vi "Collision test full.vi"(5 "Triangle to test":T1, 6 "Query triangles":T1[](array[typedef]), 7 "Octree for query triangles":T2[](array[typedef])) -> (0 "Collision point(s)":sgl[][](array[numeric]), 1 "Minimum separation vector\n(from test triangle)":sgl[](array[numeric]), 2 "Minimum separation":sgl, 3 "Indices of possible triangles":i32[](array[numeric]), 4 "Collision(s)?":bool)   [LabVIEW 2014]
doc: "This VI returns all the collision points between the test triangle and the query triangles, as well as the minimum separation vector and distance in the case of no collision."
uses:
  Typedefs/Triangle.ctl
  Typedefs/TreeNodeBox.ctl
  Typedefs/Quad.ctl
panel:
  # "PN 03/02/2015"
  # "Vertices"
  # "Edges"
  # "Unit normal"
  # "Edge unit normals"
  # "Vertices"
  # "Edges"
  # "Unit normal"
  # "Edge unit normals"
  # "Vertices"
  # "Edges"
  # "Unit normal"
  # "Edge unit normals"
  # "Vertices"
  # "Edges"
  # "Unit normal"
  # "Edge unit normals"
  # "Vertices"
  # "Edges"
  # "Unit normal"
  # "Edge unit normals"
  # "Vertices"
  # "Edges"
  # "Unit normal"
  # "Edge unit normals"
  # "Vertices"
  # "Edges"
  # "Unit normal"
  # "Edge unit normals"
  # "Vertices"
  # "Edges"
  # "Unit normal"
  # "Edge unit normals"
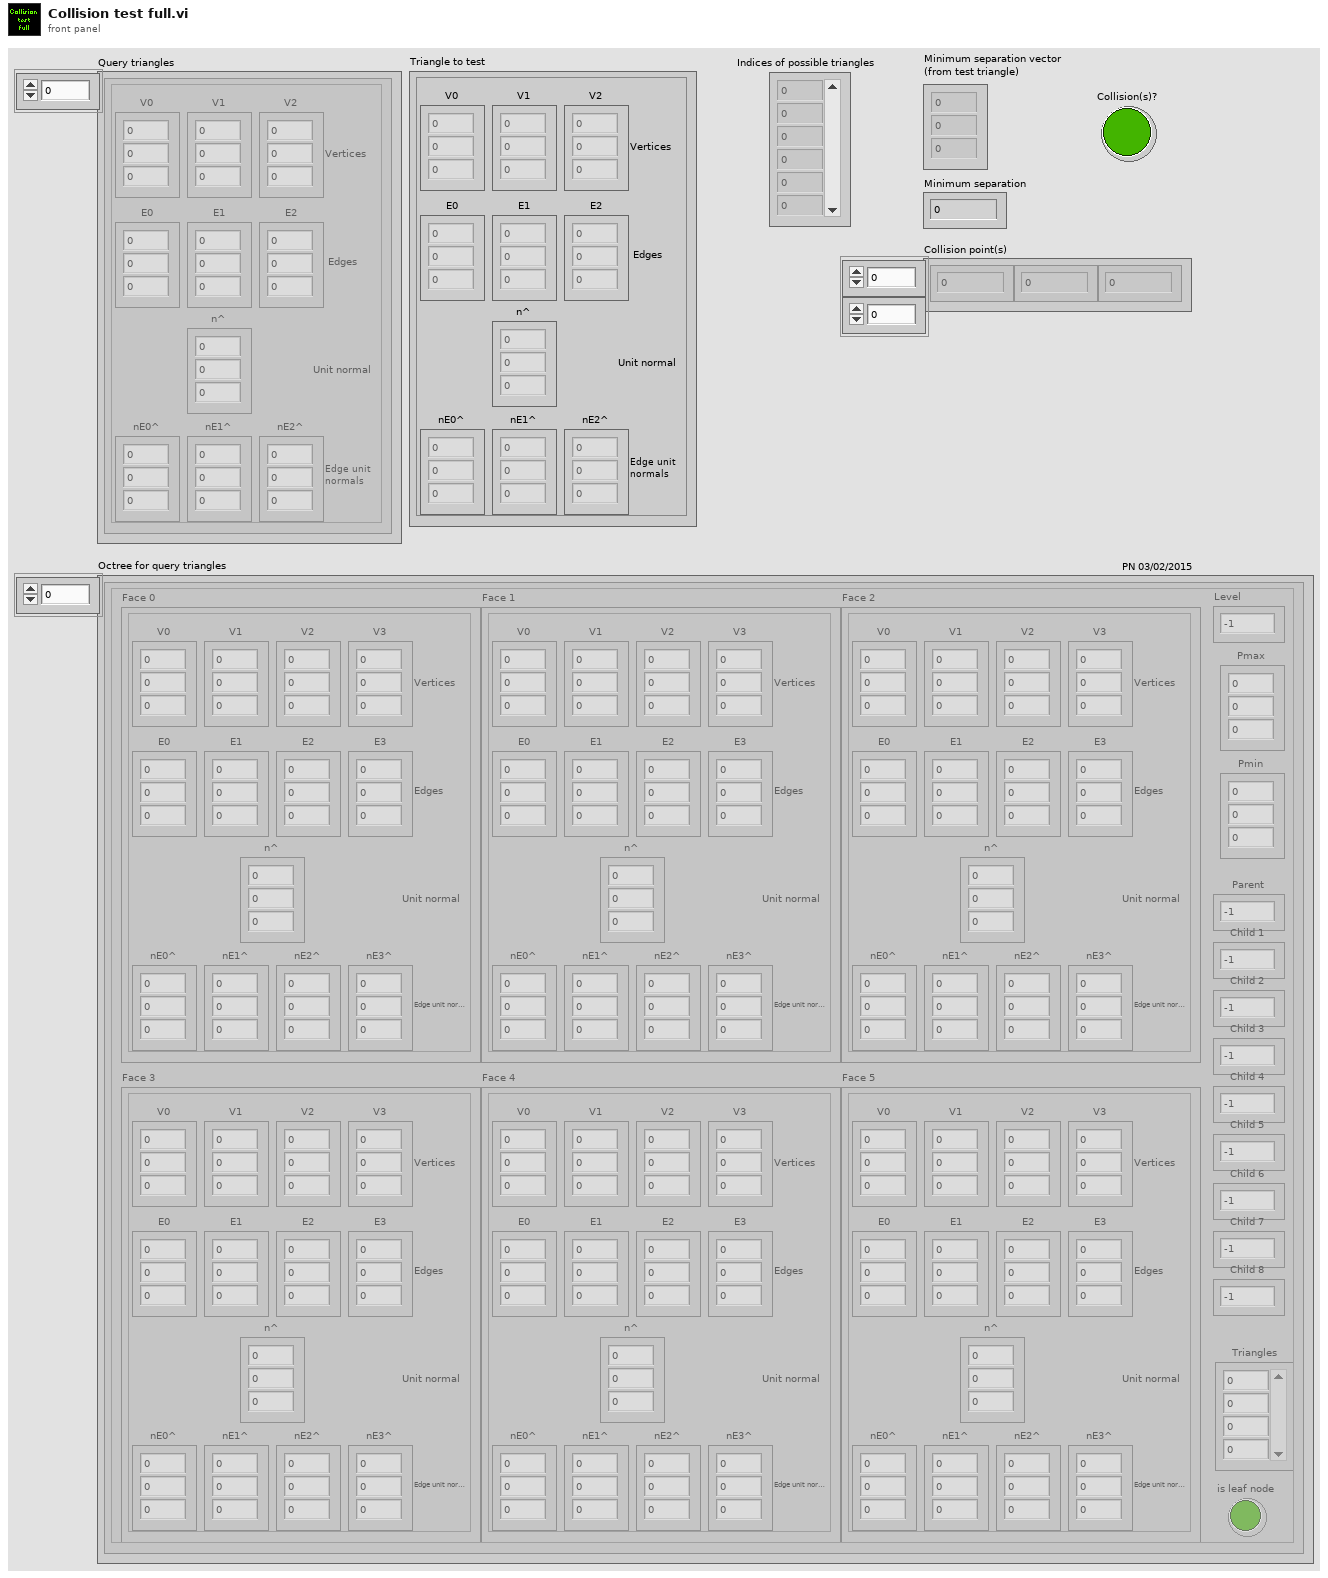
[diagram p1: front panel]
types:
  T1 = typedef "Triangle.ctl" = cluster{"V0":sgl[], "V1":sgl[], "V2":sgl[], "E0":sgl[], "E1":sgl[], "E2":sgl[], "n^":sgl[], "nE0^":sgl[], "nE1^":sgl[], "nE2^":sgl[]}
  T2 = typedef "TreeNodeBox.ctl" = cluster{"Face 0":T3, "Face 1":T3, "Face 2":T3, "Face 3":T3, "Face 4":T3, "Face 5":T3, "Level":i32, "Pmax":sgl[], "Pmin":sgl[], "Parent":i32, "Child 1":i32, "Child 2":i32, "Child 3":i32, "Child 4":i32, "Child 5":i32, "Child 6":i32, "Child 7":i32, "Child 8":i32, "Triangles":i32[], "is leaf node":bool}
  T3 = typedef "Quad.ctl" = cluster{"V0":sgl[], "V1":sgl[], "V2":sgl[], "V3":sgl[], "E0":sgl[], "E1":sgl[], "E2":sgl[], "E3":sgl[], "n^":sgl[], "nE0^":sgl[], "nE1^":sgl[], "nE2^":sgl[], "nE3^":sgl[]}
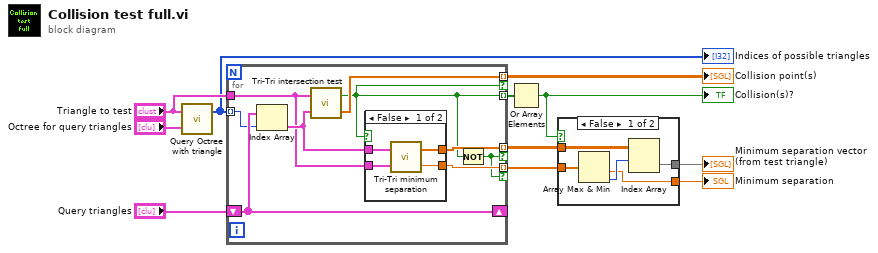
[diagram p0: block diagram]
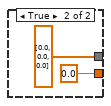
[diagram p2: hidden frame]
diagram:
  n1 = call "Query Octree with triangle.vi"("Octree node array"="Octree for query triangles", "Triangle"="Triangle to test") -> ("Indices of possible triangles"=w9:i32[])  [unwired: 1 out]
  "Indices of possible triangles" <- w9
  n2 = for {
    tunnel: "Triangle to test" -> [w15]
    tunnel: w9 -> [w19] mode=indexing
    shift-right: [w20] -> _
    shift-left: "Query triangles" -> [w20]
    tunnel: [w13] -> w7 mode=indexing
    tunnel: [w18] -> w6 mode=indexing if=w12
    tunnel: [w17] -> w1 mode=indexing if=w13
    tunnel: [w14] -> w5 mode=indexing if=w12
    n3 = Index Array(array=w20, index=w19) -> (element=w16:T1)
    n4 = call "Tri-Tri intersection test.vi"("Triangle 2"=w16, "Triangle 1"=w15) -> ("Intersection point"=w17:sgl[], "Intersection"=w13:bool)
    n5 = case shown="False" w13 {
      tunnel: w15 -> [w24 _]
      tunnel: w16 -> [w23 _]
      tunnel: [w22 _] -> w18
      tunnel: [w21 _] -> w14
      frame False {
        n6 = call "Tri-Tri minimum separation.vi"("Triangle 2"=w24, "Triangle 1"=w23) -> ("Minimum separation distance"=w22:sgl, "Minimum separation vector\nfrom triangle 2 to triange 1"=w21:sgl[])
      }
      frame True {
      }
    }
    n7 = Not(x=w13) -> (.not. x?=w12:bool)
  }
  "Collision point(s)" <- w1
  n8 = Or Array Elements(Boolean array=w7) -> (logical OR=w3:bool)
  "Collision(s)?" <- w3
  n9 = case shown="False" w3 {
    tunnel: w6 -> [w29 _]
    tunnel: w5 -> [w28 _]
    tunnel: [w26 sgl[] [0.0, 0.0, 0.0] ("Minimum separation vector\nfrom triangle 2 to triange 1")] -> w2
    tunnel: [w25 sgl 0.0] -> w4
    frame False {
      n10 = Array Max & Min(array=w29) -> (min value=w25:sgl, min index (indices)=w27:i32)  [unwired: 2 out]
      n11 = Index Array(array=w28, index (row)=w27) -> (element=w26:sgl[])  [unwired: 1 in]
    }
    frame True {
    }
  }
  "Minimum separation" <- w4
  "Minimum separation vector\n(from test triangle)" <- w2
